vi "Digital data acquired.vi"(8 "error in":errorcluster, 10 "Data":bool[](array[boolean]), 11 "Module ID":i32=-1) -> (0 "error out":errorcluster)   [LabVIEW 2020, in "NI DAQ.lvlib"]
doc: "<b>Note</b>: This VI was renamed by the DQMH Rename Event utility. Make sure the VI Description is updated to reflect the new event name, then delete this comment.\n\nBroadcasts data aqcuired from a digital or analog channel.\n_____\nCreated using DQMH Event Scripter 6.1.0.128."
uses:
  NI DAQ.lvlib
  Digital data acquired Argument--cluster.ctl
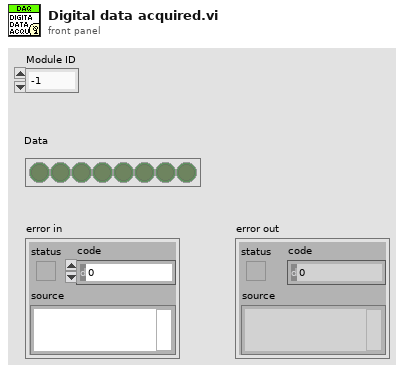
[diagram p1: front panel]
types:
  T1 = typedef "NI DAQ.lvlib/Digital data acquired Argument--cluster.ctl" = cluster{"Module ID":i32, "Data":bool[]}
  T2 = typedef "NI DAQ.lvlib/Broadcast Events--cluster.ctl" = cluster{"Module Did Init":refnum<user-event>, "Status Updated":refnum<user-event>, "Error Reported":refnum<user-event>, "Module Did Stop":refnum<user-event>, "Update Module Execution Status":refnum<user-event>, "Digital data acquired":refnum<user-event>, "Device connected":refnum<user-event>, "Connection failed":refnum<user-event>, "Analog data acquired":refnum<user-event>}
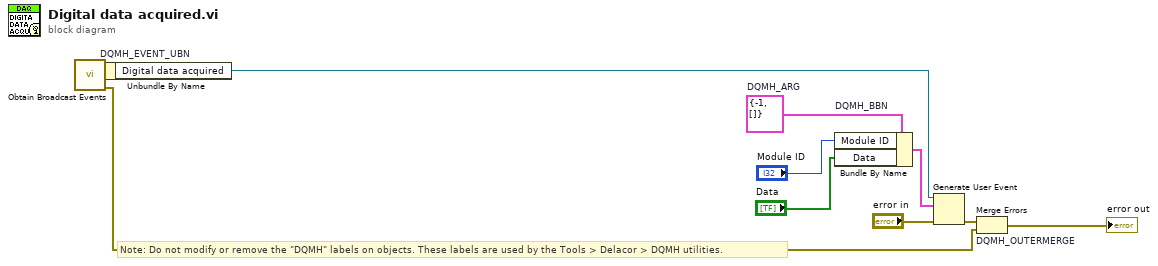
[diagram p0: block diagram]
diagram:
  w5 = T1 {"Module ID"=-1, "Data"=[]}  # DQMH_ARG
  # "Note: Do not modify or remove the \"DQMH\" labels on objects. These labels are used by the Tools > Delacor > DQMH utilities."
  n1 = call "Obtain Broadcast Events.vi"() -> ("error out"=w3:errorcluster, "NI DAQ Broadcast Events"=w2:T2)  [unwired: 10 in]
  n2 = Unbundle By Name "DQMH_EVENT_UBN"(w2) -> ("Digital data acquired"=w7:refnum<user-event>)
  n3 = Bundle By Name "DQMH_BBN"(cluster=w5, "Module ID"="Module ID", "Data"="Data") -> (w8:T1)
  n4 = Generate User Event(user event=w7, event data cluster=w8, error in="error in") -> (error out=w6:errorcluster)  [unwired: 1 in, 1 out]
  n5 = Merge Errors "DQMH_OUTERMERGE"(w6, w3) -> (→"error out":errorcluster)
